vi "set Volume Index And Time.vi"(9 "pVolumeTimeInSeconds":dbl, 10 "pVolumeIndex":i32, 11 "pSinkId":i32) -> (3 "function return":i32)   [LabVIEW 2012, in "cvlib.lvlib"]
doc: "extern \"C\"__declspec(dllexport) long __cdecl setVolumeIndexAndTime( long pSinkId,\n long pVolumeIndex,\n double pVolumeTimeInSeconds);"
uses:
  cvlib.lvlib
  cvlib.dll
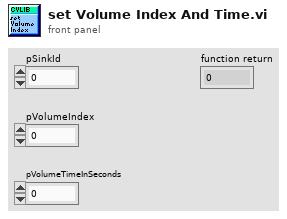
[diagram p1: front panel]
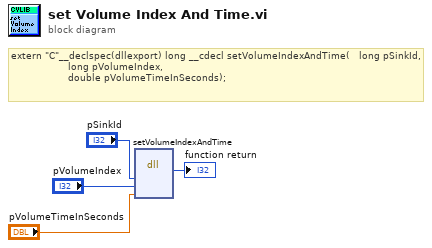
[diagram p0: block diagram]
diagram:
  # "extern \"C\"__declspec(dllexport) long __cdecl setVolumeIndexAndTime( \t\tlong pSinkId,\n\t\t\t\t\t\t\t\t\t\t\t\t\t\t\t\t\t\t\tlong pVolumeIndex,\n\t\t\t\t\t\t\t\t\t\t\t\t\t\t\t\t\t\t\tdouble pVolumeTimeInSeconds);"
  n1 = dll-call lib="C:/Users/myerslab/workspace2/Libraries/ClearVolume/cpp/labview/lvcvlib/cvlib.*" fn="setVolumeIndexAndTime"("pSinkId"="pSinkId", "pVolumeIndex"="pVolumeIndex", "pVolumeTimeInSeconds"="pVolumeTimeInSeconds") -> (→"function return":i32)  [unwired: 6 in, 2 out]
